vi "Rabi.vi"() -> ()   [LabVIEW 2017]
panel:
  out "IsVisible":bool
  in  "CodeDir":path
  in  "Selected File":u16(ring)
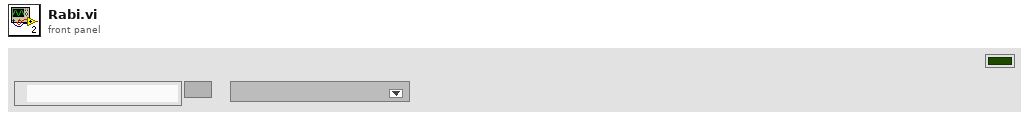
[diagram p1: front panel]
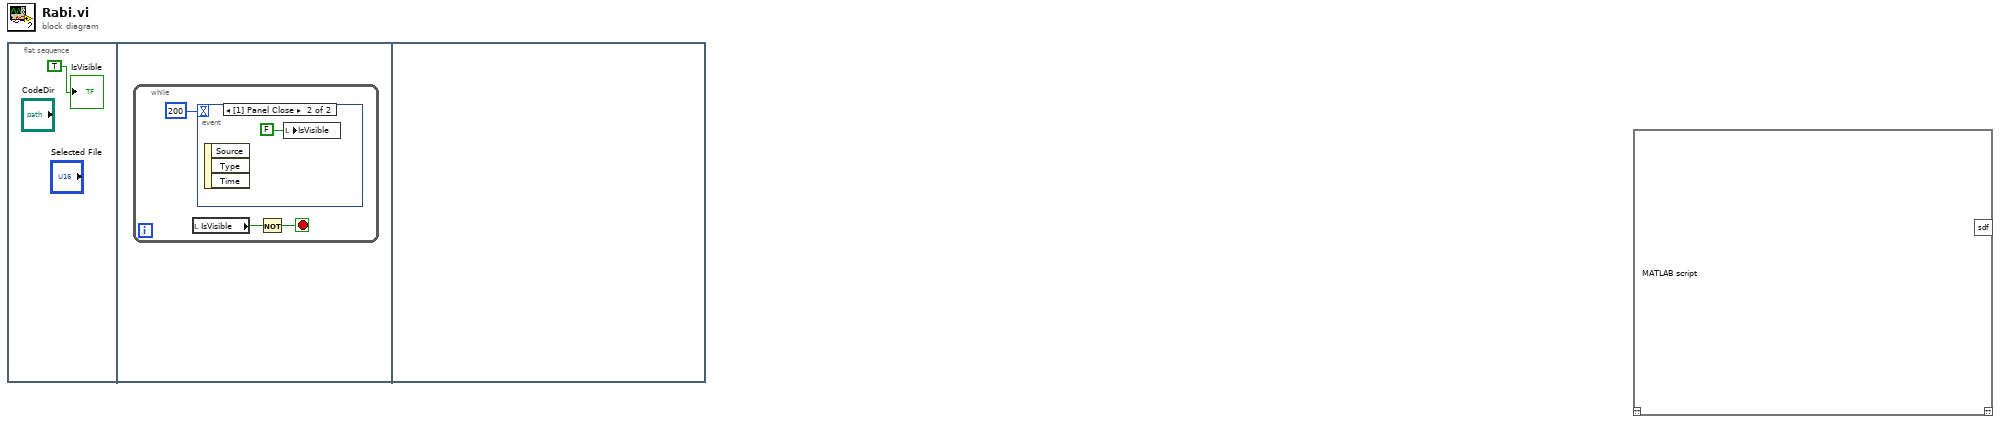
[diagram p0: block diagram]
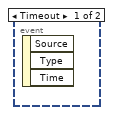
[diagram p2: hidden frame]
diagram:
  n1 = flat-sequence {
    frame #0 {
      "IsVisible" <- TRUE ("IsVisible")
    }
    frame #1 {
      n2 = while {
        stop <- w2 stop-if-true
        n3 = local read "IsVisible"() -> (w3:bool)
        n4 = event shown="[1] Panel Close" {
          selector: _ -> [_ _]
          dyn-events: _ -> [_ _]
          timeout: 200 -> [_ _]
          event Timeout {
            n5 = event-data() -> ()  [unwired: 1 in, 3 out]
          }
          event Panel Close {
            n6 = event-data() -> ()  [unwired: 1 in, 3 out]
            n7 = local write "IsVisible"(FALSE ("IsVisible")) -> ()
          }
        }
        n8 = Not(x=w3) -> (.not. x?=w2:bool)
      }
    }
    frame #2 {
    }
  }
  n9 = script code="MATLAB script"() -> ()  [unwired: 1 in, 2 out]
